vi "DEBUG_GET_REFNUM.vi"(8 "error in":errorcluster, 11 "BigMAQ in":refnum<class "BigMAQ.lvclass">) -> (0 "error out":errorcluster, 2 "IMAQ REFNUMS":T1[](array[typedef]), 3 "BigMAQ out":refnum<class "BigMAQ.lvclass">)   [LabVIEW 2019, in "BigMAQ.lvclass"]
uses:
  BigMAQ.lvclass
  <vilib>/vision/Image Controls.llb/IMAQ Image.ctl
  BigMAQ.lvclass/BigMAQ.ctl
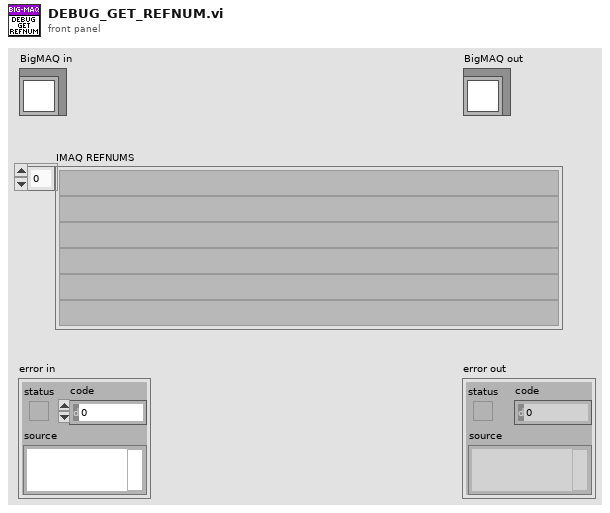
[diagram p1: front panel]
types:
  T1 = typedef "IMAQ Image.ctl" = refnum<image>
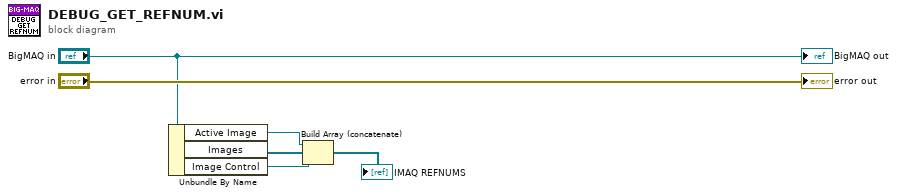
[diagram p0: block diagram]
diagram:
  n1 = Unbundle By Name("BigMAQ in") -> ("Active Image"=w4:T1, "Images"=w3:T1[], "Image Control"=w2:T1)
  n2 = Build Array (concatenate)(w4, w3, w2) -> (→"IMAQ REFNUMS":T1[])
  "error out" <- "error in"
  "BigMAQ out" <- "BigMAQ in"
